vi "TachDataGcode_PosToQueue.vi"(8 "error in (no error)":errorcluster, 9 "OUTDGREES":cluster{"A":dbl, "B":dbl}, 10 "outPOS":T1, 11 "queue out":refnum<queue>) -> (0 "error out":errorcluster)   [LabVIEW 2017]
uses:
  libraryGcode/control/UartCmdQueueUpdate.ctl
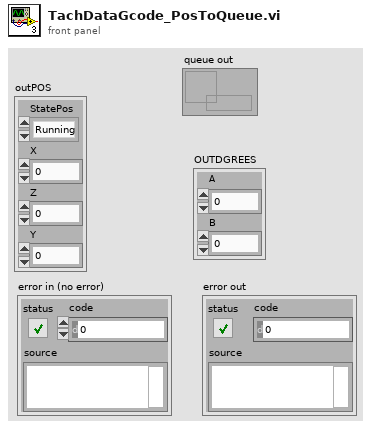
[diagram p1: front panel]
types:
  T1 = cluster{"StatePos":enum16{"Running", "Waiting", "Pos", "IDLE"}, "X":dbl, "Z":dbl, "Y":dbl}
  T2 = typedef "UartCmdQueueUpdate.ctl" = enum16{"updatePos", "UpdateConfigAccel", "UpdateConfigFeed", "UpdateConfigUnit", "UpdateConfigStartAccel"}
  T3 = cluster{"Command":T2, cluster{"X":dbl, "Z":dbl, "Y":dbl}, "OUTDGREES":cluster{"A":dbl, "B":dbl}}
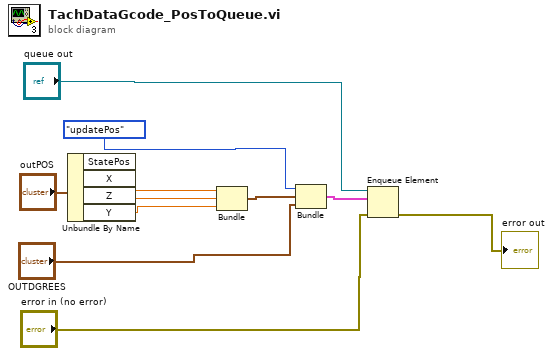
[diagram p0: block diagram]
diagram:
  n1 = Unbundle By Name("outPOS") -> ("X"=w3:dbl, "Z"=w8:dbl, "Y"=w4:dbl)  [unwired: 1 out]
  n2 = Bundle("X"=w3, "Z"=w8, "Y"=w4) -> (w9:cluster{"X":dbl, "Z":dbl, "Y":dbl})  [unwired: 1 in]
  n3 = Bundle("Command"=UartCmdQueueUpdate."updatePos", w9, "OUTDGREES"="OUTDGREES") -> (w11:T3)  [unwired: 1 in]
  n4 = Enqueue Element(queue="queue out", element=w11, error in (no error)="error in (no error)") -> (error out=→"error out":errorcluster)  [unwired: 1 in, 2 out]
